vi "Find DLP Device COMs.vi"(6 "error in (no error)":errorcluster) -> (0 "error out":errorcluster, 3 "DLP COMs":T1(array[cluster]))   [LabVIEW 2020, in "DLP Design Modules Driver.lvlib"]
uses:
  <vilib>/Instr/_visa.llb/VISA Find Search Mode.ctl
  <vilib>/Instr/_visa.llb/VISA Configure Serial Port (Instr).vi
  DLP Design Modules Driver.lvlib
panel:
  in  "Tab Control":enum32{"Page 1", "Page 2"}(tab)
  out "COM List":string[](array[string])
  out "Ping Responses":string[](array[string])
  out "Read Buffer":string
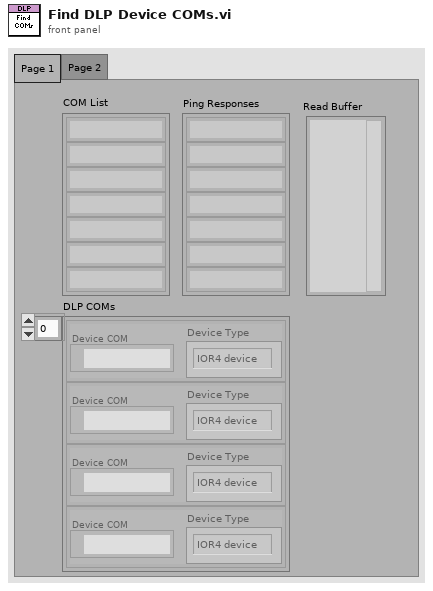
[diagram p1: front panel]
types:
  T1 = cluster{"Device COM":refnum<visa-resource-name>, "Device Type":enum16{"IOR4 device", "IO20 device"}}[]
  T2 = cluster{"VISA resource name":refnum<visa-resource-name>, "Device Type":enum16{"IOR4 device", "IO20 device"}}[]
  T3 = typedef "VISA Find Search Mode.ctl" = u32
  T4 = cluster{"VISA resource name out":refnum<visa-resource-name>, "Device Type":enum16{"IOR4 device", "IO20 device"}}
  T5 = cluster{"VISA resource name out":refnum<visa-resource-name>, "Device Type":enum16{"IOR4 device", "IO20 device"}}[]
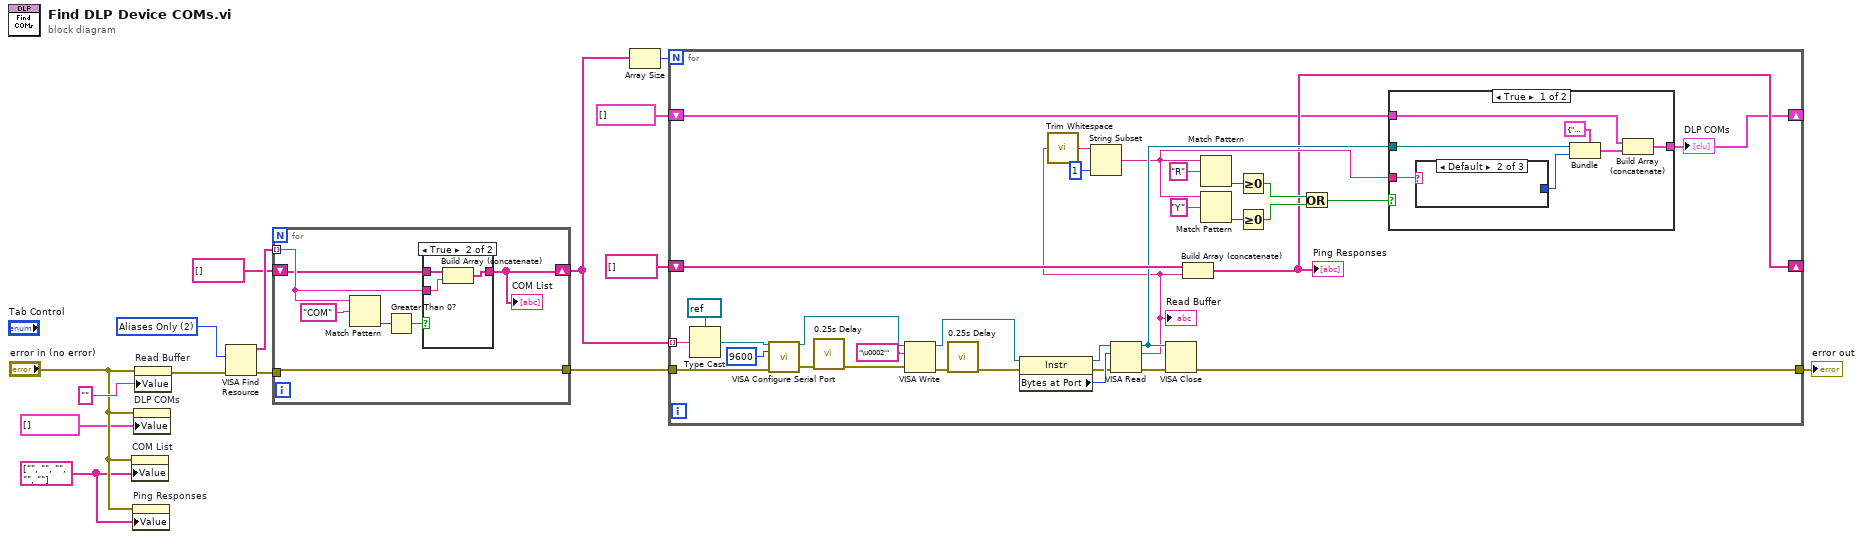
[diagram p0: block diagram]
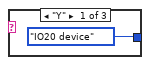
[diagram p2: hidden frame]
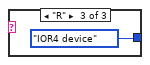
[diagram p3: hidden frame]
diagram:
  w7 = string[] ["", "", "", "", ""] ("Ping Response")
  w15 = T3 2 items=["Canonical Names Only"=0, "Aliases Only"=2, "Include Matching Aliases"=3, "Include All Aliases"=4] ("Search Mode")
  n1 = property on="COM List" class="Arr (strict)"(error in="error in (no error)", "Value"=w7) -> ()  [unwired: 1 in, 2 out]
  n2 = property on="Ping Responses" class="Arr (strict)"(error in="error in (no error)", "Value"=w7) -> ()  [unwired: 1 in, 2 out]
  n3 = property on="DLP COMs" class="Arr (strict)"(error in="error in (no error)", "Value"=T2 [] ("DLP COMs")) -> ()  [unwired: 1 in, 2 out]
  n4 = property on="Read Buffer" class="Str"(error in="error in (no error)", "Value"="" ("Read Buffer")) -> (error out=w5:errorcluster)  [unwired: 1 in, 1 out]
  n5 = VISA Find Resource(8:w5, 10:w15) -> (0:w6:errorcluster, 3:w14:string[])  [unwired: 1 in, 1 out]
  n6 = for {
    tunnel: w14 -> [w19] mode=indexing
    shift-right: [w18] -> w4
    shift-left: string[] [] -> [w17]
    tunnel: [w16] -> w10
    tunnel: w6 -> [w16]
    n7 = Match Pattern(string=w19, regular expression="COM") -> (offset past match=w21:i32)  [unwired: 1 in, 3 out]
    n8 = Greater Than 0?(x=w21) -> (x > 0?=w20:bool)
    n9 = case shown="True" w20 {
      tunnel: w19 -> [_ w26]
      tunnel: [w23 w25] -> w18
      tunnel: w17 -> [w23 w24]
      frame False {
      }
      frame True {
        n10 = Build Array (concatenate)(w24, w26) -> (w25:string[])
      }
    }
    "COM List" <- w18
  }
  n11 = Array Size(array=w4) -> (size(s)=w3:i32)
  n12 = for {
    N: w3 -> [_]
    tunnel: w4 -> [w48] mode=indexing
    tunnel: w10 -> [w53]
    shift-right: [w33] -> _
    shift-left: string[] [] -> [w46]
    tunnel: [w30] -> w9
    shift-right: [w31] -> _
    shift-left: T2 [] ("DLP COMs") -> [w32]
    n13 = Type Cast(type=refnum<visa-resource-name> refnum ("VISA resource name"), x=w48) -> (*(type *) &x=w54:refnum<visa-resource-name>)
    n14 = call-poly "VISA Configure Serial Port"("VISA resource name"=w54, "baud rate (9600)"=u32 9600, "error in (no error)"=w53) -> ("VISA resource name out"=w27:refnum<visa-resource-name>, "error out"=w29:errorcluster)  [unwired: 11 in]
    n15 = call "0.25s Delay"("error in (no error)"=w29) -> ("error out"=w28:errorcluster)  [unwired: 10 in]
    n16 = VISA Write(VISA resource name=w27, write buffer="\u0002'", error in (no error)=w28) -> (VISA resource name out=w47:refnum<visa-resource-name>, error out=w44:errorcluster)  [unwired: 1 out]
    n17 = call "0.25s Delay"("error in (no error)"=w44) -> ("error out"=w43:errorcluster)  [unwired: 10 in]
    n18 = property class="Instr"(reference=w47, error in=w43) -> (reference out=w58:refnum<visa-resource-name>, error out=w56:errorcluster, "Bytes at Port"=w57:u32)
    n19 = VISA Read(VISA resource name=w58, byte count=w57, error in (no error)=w56) -> (VISA resource name out=w45:refnum<visa-resource-name>, read buffer=w39:string, error out=w59:errorcluster)  [unwired: 1 out]
    "Read Buffer" <- w39
    n20 = call <vilib>:"Trim Whitespace.vi"("string"=w39) -> ("trimmed string"=w41:string)  [unwired: 1 in]
    n21 = String Subset(string=w41, length (rest)=1 ("length (rest)")) -> (substring=w34:string)  [unwired: 1 in]
    n22 = VISA Close(VISA resource name=w45, error in (no error)=w59) -> (error out=w30:errorcluster)
    n23 = Build Array (concatenate)(w46, w39) -> (w33:string[])
    "Ping Responses" <- w33
    n24 = Match Pattern(string=w34, regular expression="R") -> (offset past match=w49:i32)  [unwired: 1 in, 3 out]
    n25 = Match Pattern(string=w34, regular expression="Y") -> (offset past match=w51:i32)  [unwired: 1 in, 3 out]
    n26 = Greater Or Equal To 0?(x=w49) -> (x >= 0?=w35:bool)
    n27 = Greater Or Equal To 0?(x=w51) -> (x >= 0?=w37:bool)
    n28 = Or(x=w35, y=w37) -> (x .or. y?=w36:bool)
    n29 = case shown="True" w36 {
      tunnel: w45 -> [w66 _]
      tunnel: [w63 w69] -> w31
      tunnel: w34 -> [w65 _]
      tunnel: w32 -> [w64 w69]
      frame True {
        n30 = case shown="Default" w65 {
          tunnel: [enum16{"IOR4 device", "IO20 device"}."IO20 device" ("Device Type") _ enum16{"IOR4 device", "IO20 device"}."IOR4 device" ("Device Type")] -> w62
          frame "Y" {
          }
          frame Default {
          }
          frame "R" {
          }
        }
        n31 = Bundle(cluster=T4 {"VISA resource name out"="", "Device Type"=enum."IOR4 device"}, "VISA resource name out"=w66, "Device Type"=w62) -> (w61:T4)
        n32 = Build Array (concatenate)(w64, w61) -> (w63:T5)
      }
      frame False {
      }
    }
    "DLP COMs" <- w31
  }
  "error out" <- w9
